vi "XYStage_Initialize_ASI_MS2000.vi"(8 "error in (no error)":errorcluster, 11 "VISA resource name":refnum<visa-resource-name>) -> (0 "error out":errorcluster, 3 "VISA resource name out":refnum<visa-resource-name>)   [LabVIEW 2013]
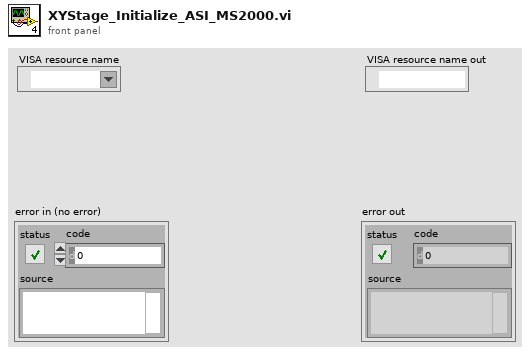
[diagram p1: front panel]
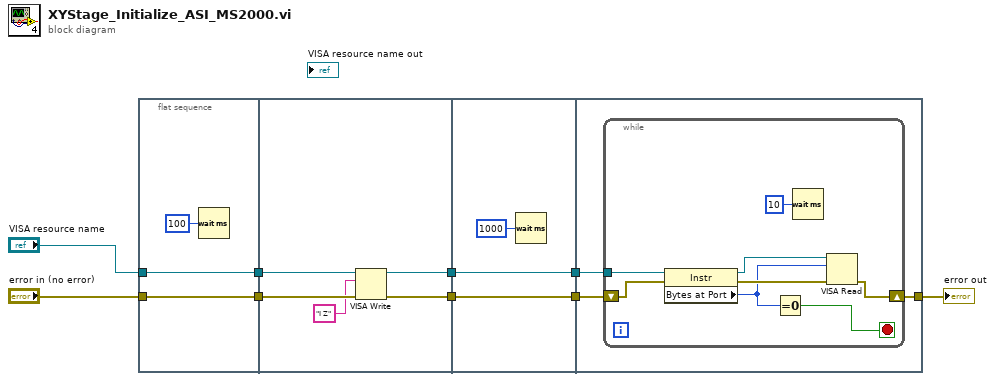
[diagram p0: block diagram]
diagram:
  n1 = flat-sequence {
    tunnel: "error in (no error)" -> [w12]
    tunnel: [w12] -> w8
    tunnel: "VISA resource name" -> [w10]
    tunnel: [w10] -> w5
    tunnel: w8 -> [w17]
    tunnel: [w16] -> w7
    tunnel: w5 -> [w15]
    tunnel: [w13] -> w3
    tunnel: w7 -> [w20]
    tunnel: [w20] -> w6
    tunnel: w3 -> [w18]
    tunnel: [w18] -> w2
    tunnel: w6 -> [w22]
    tunnel: w2 -> [w23]
    tunnel: [w21] -> w1
    frame #0 {
      n2 = Wait (ms)(milliseconds to wait=u32 100) -> ()  [unwired: 1 out]
    }
    frame #1 {
      n3 = VISA Write(VISA resource name=w15, write buffer="I Z", error in (no error)=w17) -> (VISA resource name out=w13:refnum<visa-resource-name>, error out=w16:errorcluster)  [unwired: 1 out]
    }
    frame #2 {
      n4 = Wait (ms)(milliseconds to wait=u32 1000) -> ()  [unwired: 1 out]
    }
    frame #3 {
      n5 = while {
        tunnel: w23 -> [w31]
        shift-right: [w25] -> w21
        shift-left: w22 -> [w30]
        stop <- w29 stop-if-true
        n6 = property class="Instr"(reference=w31, error in=w30) -> (reference out=w26:refnum<visa-resource-name>, error out=w28:errorcluster, "Bytes at Port"=w27:u32)
        n7 = Equal To 0?(x=w27) -> (x = 0?=w29:bool)
        n8 = Wait (ms)(milliseconds to wait=u32 10) -> ()  [unwired: 1 out]
        n9 = VISA Read(VISA resource name=w26, byte count=w27, error in (no error)=w28) -> (error out=w25:errorcluster)  [unwired: 3 out]
      }
    }
  }
  "error out" <- w1
